vi "FGV Project Name.vi"(11 "Project Name":string) -> (3 "Project Name Out":string)   [LabVIEW 2020, in "Panter Dashboard.lvlib"]
uses:
  Panter Dashboard.lvlib
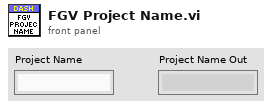
[diagram p1: front panel]
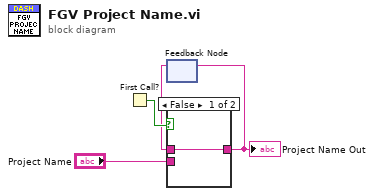
[diagram p0: block diagram]
diagram:
  n1 = First Call?() -> (First Call?: T/F=w4:bool)
  n2 = feedback #1() -> (w1:string)  [unwired: 1 in]
  n3 = case shown="False" w4 {
    tunnel: "Project Name" -> [_ w6]
    tunnel: [w5 w6] -> w2
    tunnel: w1 -> [w5 _]
    frame False {
    }
    frame True {
    }
  }
  "Project Name Out" <- w2
  n4 = feedback-in #1(w2) -> ()
